vi "FIB HV target match.vi"(11 "Capella HV Data Output":T3 {"Column Vac (Torr)" format="%.2e"; "Gun Vac (Torr)" format="%.2e"; "Lens2 Actual (V)" format="%.1f"; "Lens1 Actual (V)" format="%.1f"; "Emission Actual (uA)" format="%.3f"; "Extrator Actual (V)" format="%.1f"; "Tip Lifetime (uAhr)" format="%.2f"; "Lens2 Target (V)" format="%.1f"; "Lens1 Target (V)" format="%.1f"; "SuppI (uA)" format="%.3f"; "Suppressor (V)" format="%.1f"; "Emission Target (uA)" format="%.3f"; "Extrator Target (V)" format="%.1f"; "Accelerator Actual (V)" format="%.1f"; "Accelerator Target (V)" format="%.1f"; "Filament (A)" format="%.2f"}) -> (0 "Max relative error (%)":sgl format="%.1f", 1 "Relative Error (%)":T1 {"Lens2 Error" format="%.1f"; "Lens1 Error" format="%.1f"; "Extrator Error" format="%.1f"; "Accelerator Error" format="%.1f"}, 2 "Max absolute error (V)":sgl, 3 "Absolue Error (V)":T2 {"Lens2 Error (V)" format="%.1f"; "Lens1 Error (V)" format="%.1f"; "Extrator Error (V)" format="%.1f"; "Accelerator Error (V)" format="%.1f"}, 4 "Min relative error (%)":sgl format="%.1f", 6 "Mean relative error (%)":sgl format="%.1f")   [LabVIEW 2018]
uses:
  <vilib>/Analysis/baseanly.llb/Mean (DBL).vi
  <vilib>/Analysis/NI_AALBase.lvlib
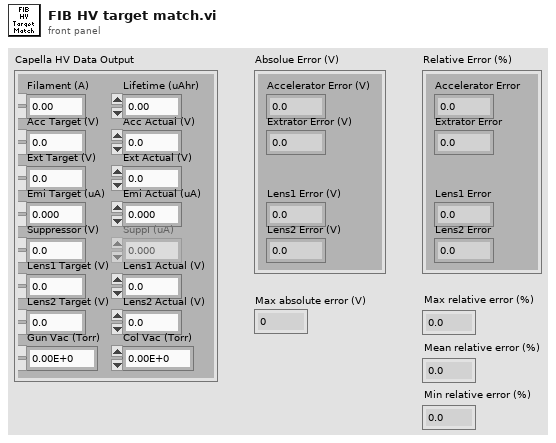
[diagram p1: front panel]
types:
  T1 = cluster{"Accelerator Error":sgl, "Extrator Error":sgl, "Lens1 Error":sgl, "Lens2 Error":sgl}
  T2 = cluster{"Accelerator Error (V)":sgl, "Extrator Error (V)":sgl, "Lens1 Error (V)":sgl, "Lens2 Error (V)":sgl}
  T3 = cluster{"Filament (A)":sgl, "Accelerator Target (V)":sgl, "Accelerator Actual (V)":sgl, "Extrator Target (V)":sgl, "Extrator Actual (V)":sgl, "Emission Target (uA)":sgl, "Emission Actual (uA)":sgl, "Suppressor (V)":sgl, "SuppI (uA)":sgl, "Lens1 Target (V)":sgl, "Lens1 Actual (V)":sgl, "Lens2 Target (V)":sgl, "Lens2 Actual (V)":sgl, "Gun Vac (Torr)":sgl, "Column Vac (Torr)":sgl, "Tip Lifetime (uAhr)":sgl}
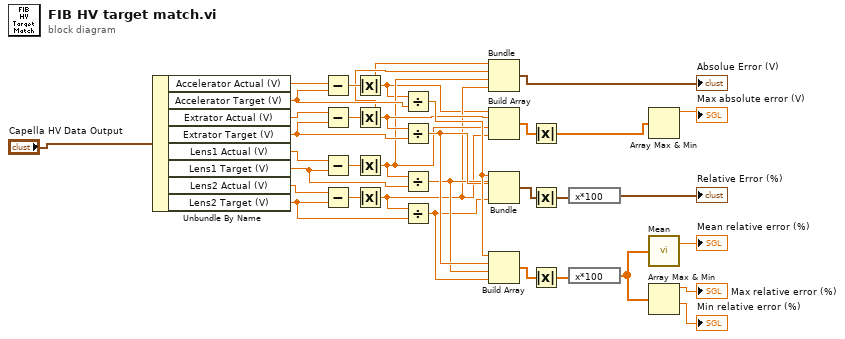
[diagram p0: block diagram]
diagram:
  n1 = Unbundle By Name("Capella HV Data Output") -> ("Accelerator Actual (V)"=w32:sgl, "Accelerator Target (V)"=w31:sgl, "Extrator Actual (V)"=w29:sgl, "Extrator Target (V)"=w28:sgl, "Lens1 Actual (V)"=w25:sgl, "Lens1 Target (V)"=w24:sgl, "Lens2 Actual (V)"=w23:sgl, "Lens2 Target (V)"=w22:sgl)
  n2 = Subtract(x=w32, y=w31) -> (x-y=w33:sgl)
  n3 = Subtract(x=w29, y=w28) -> (x-y=w30:sgl)
  n4 = Subtract(x=w25, y=w24) -> (x-y=w26:sgl)
  n5 = Subtract(x=w23, y=w22) -> (x-y=w27:sgl)
  n6 = Absolute Value(x=w33) -> (abs(x)=w3:sgl)
  n7 = Absolute Value(x=w30) -> (abs(x)=w6:sgl)
  n8 = Absolute Value(x=w26) -> (abs(x)=w5:sgl)
  n9 = Absolute Value(x=w27) -> (abs(x)=w4:sgl)
  n10 = Divide(x=w3, y=w31) -> (x/y=w19:sgl)
  n11 = Divide(x=w6, y=w28) -> (x/y=w18:sgl)
  n12 = Divide(x=w5, y=w24) -> (x/y=w17:sgl)
  n13 = Divide(x=w4, y=w22) -> (x/y=w16:sgl)
  n14 = Bundle(w3, w6, w5, w4) -> (→"Absolue Error (V)":cluster{sgl, sgl, sgl, sgl})  [unwired: 1 in]
  n15 = Build Array(w3, w6, w5, w4) -> (w7:sgl[])
  n16 = Bundle(w19, w18, w17, w16) -> (w9:cluster{sgl, sgl, sgl, sgl})  [unwired: 1 in]
  n17 = Build Array(w19, w18, w17, w16) -> (w12:sgl[])
  n18 = Absolute Value(x=w7) -> (abs(x)=w2:sgl[])
  n19 = Absolute Value(x=w9) -> (abs(x)=w8:cluster{sgl, sgl, sgl, sgl})
  n20 = Absolute Value(x=w12) -> (abs(x)=w11:sgl[])
  n21 = expression code="x*100"(w8) -> (→"Relative Error (%)":cluster{sgl, sgl, sgl, sgl})
  n22 = expression code="x*100"(w11) -> (w10:sgl[])
  n23 = Array Max & Min(array=w2) -> (max value=→"Max absolute error (V)":sgl)  [unwired: 3 out]
  n24 = call-poly <vilib>:"Mean.vi"("X"=w10) -> ("mean"=→"Mean relative error (%)":dbl)  [unwired: 1 out]
  n25 = Array Max & Min(array=w10) -> (max value=→"Max relative error (%)":sgl, min value=→"Min relative error (%)":sgl)  [unwired: 2 out]
